vi "Configure Slew Rate.vi"   [LabVIEW 2012, in "NH Research Regenerative Test Series.lvlib"]
doc: "Sets the slew rate for all programmed changes in the output of the module. This command programs both positive and negative going slew rates. Although any slew rate value may be entered, the module selects a slew rate that is closest to the programmed value. Slew rates less than the minimum value are set to minimum. Slew rates greater than the maximum value are set to maximum."
uses:
  <instrlib>/NH Research Regenerative Test Series/NH Research Regenerative Test Series.lvlib
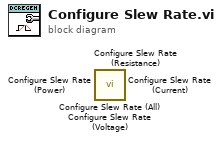
[diagram p0: block diagram]
diagram:
  n1 = call <instrlib>:"Configure Slew Rate (All).vi"() -> ()  [unwired: 14 in, 2 out]
  n2 = call <instrlib>:"Configure Slew Rate (Resistance).vi"() -> ()  [unwired: 14 in, 2 out]
  n3 = call <instrlib>:"Configure Slew Rate (Power).vi"() -> ()  [unwired: 14 in, 2 out]
  n4 = call <instrlib>:"Configure Slew Rate (Current).vi"() -> ()  [unwired: 14 in, 2 out]
  n5 = call <instrlib>:"Configure Slew Rate (Voltage).vi"() -> ()  [unwired: 14 in, 2 out]
